vi "read_ini_AdditionalSoftLimits.vi"(8 "error in (no error)":errorcluster caption="错误输入（无错误）", 10 "file ref in":T1, 11 "MotorSystem 输入":refnum<class "MotorSystem.lvclass">) -> (0 "error out":errorcluster caption="错误输出", 2 "file ref out":T1, 3 "MotorSystem 输出":refnum<class "MotorSystem.lvclass">)   [LabVIEW 2016, in "MotionControl.lvlib" / "MotorSystem.lvclass"]
uses:
  <userlib>/MotionControl/MotorSystem/MotorSystem.lvclass
  <vilib>/Utility/config.llb/Config Data RefNum.ctl
  <userlib>/MotionControl/MotorSystem/MotorSystem.lvclass/MotorSystem.ctl
  <vilib>/Utility/config.llb/Read Key (I32).vi
  <vilib>/Utility/config.llb/Read Key (String).vi
  <vilib>/Utility/config.llb/Read Key (Double).vi
  <vilib>/Utility/config.llb/NI_LVConfig.lvlib
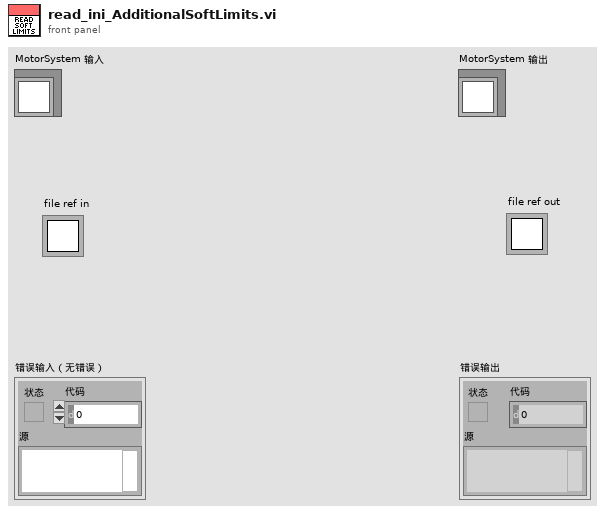
[diagram p1: front panel]
types:
  T1 = typedef "NI_LVConfig.lvlib/Config Data RefNum.ctl" = refnum<k1>
  T2 = cluster{"value":string, cluster{"value":dbl, "value":dbl}}
  T3 = cluster{cluster{"value":string, cluster{"value":dbl, "value":dbl}}[]}
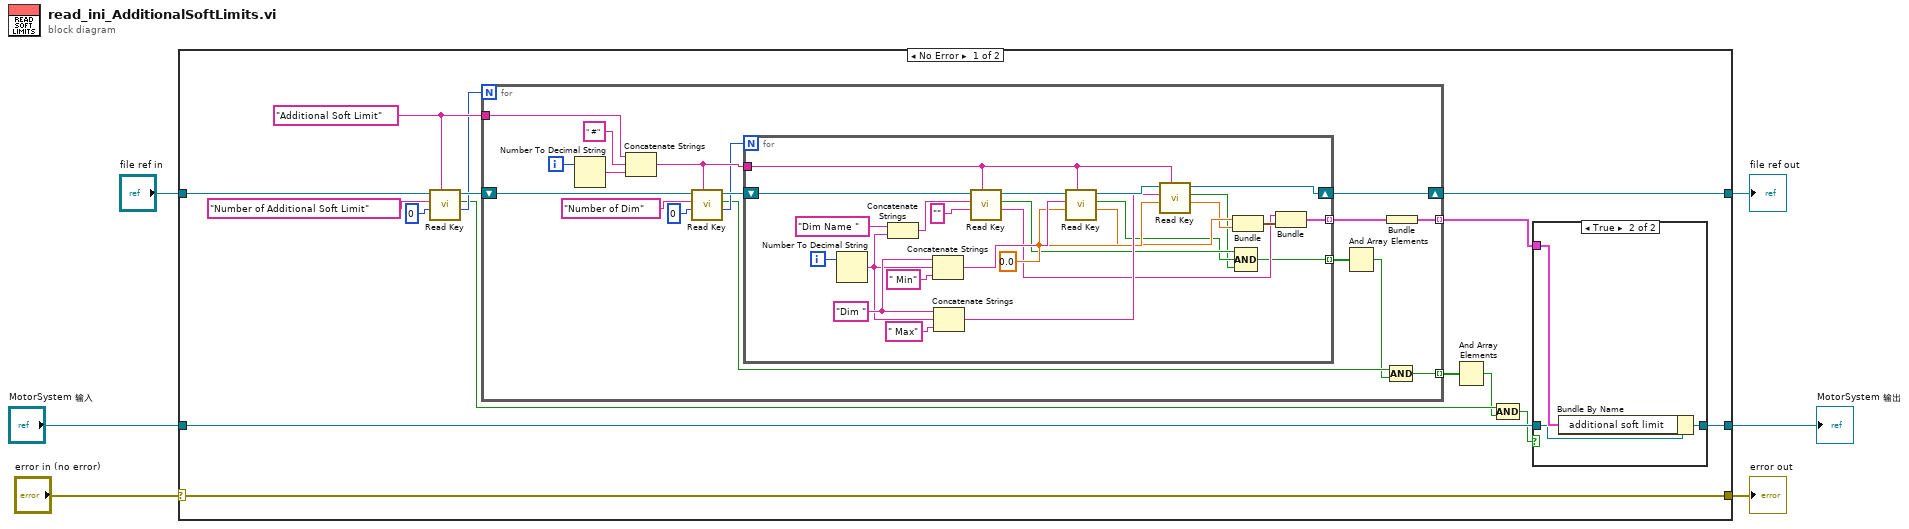
[diagram p0: block diagram]
diagram:
  n1 = case shown="No Error" "error in (no error)" {
    selector: "error in (no error)" -> [w21 w70]
    tunnel: [w21 w70] -> w5
    tunnel: [w11 w69] -> w3
    tunnel: "MotorSystem 输入" -> [w12 w69]
    tunnel: "file ref in" -> [w20 w68]
    tunnel: [w16 w68] -> w1
    frame No Error {
      w18 = "Additional Soft Limit"
      n2 = call-poly <vilib>:"Read Key.vi"("section"=w18, "default value"=0, "key"="Number of Additional Soft Limit", "refnum"=w20) -> ("value"=w14:i32, "found?"=w9:bool, "refnum out"=w17:T1)  [unwired: 4 in, 1 out]
      n3 = for {
        N: w14 -> [_]
        tunnel: w18 -> [w42]
        shift-right: [w34] -> w16
        shift-left: w17 -> [w38]
        tunnel: [w30] -> w13 mode=indexing
        tunnel: [w26] -> w10 mode=indexing
        i -> [w39]
        n4 = Number To Decimal String(number=w39) -> (decimal integer string=w40:string)  [unwired: 1 in]
        n5 = Concatenate Strings(w42, " #", w40) -> (w35:string)
        n6 = call-poly <vilib>:"Read Key.vi"("section"=w35, "default value"=0, "key"="Number of Dim", "refnum"=w38) -> ("value"=w32:i32, "found?"=w28:bool, "refnum out"=w37:T1)  [unwired: 4 in, 1 out]
        n7 = for {
          N: w32 -> [_]
          shift-right: [w54] -> w34
          shift-left: w37 -> [w67]
          tunnel: w35 -> [w55]
          tunnel: [w47] -> w31 mode=indexing
          tunnel: [w43] -> w29 mode=indexing
          i -> [w66]
          w52 = 0.0
          w59 = "Dim "
          n8 = Number To Decimal String(number=w66) -> (decimal integer string=w58:string)  [unwired: 1 in]
          n9 = Concatenate Strings("Dim Name ", w58) -> (w64:string)
          n10 = Concatenate Strings(w59, w58, " Min") -> (w61:string)
          n11 = Concatenate Strings(w59, w58, " Max") -> (w56:string)
          n12 = call-poly <vilib>:"Read Key.vi"("section"=w55, "default value"="", "key"=w64, "refnum"=w67) -> ("value"=w48:string, "found?"=w46:bool, "refnum out"=w63:T1)  [unwired: 4 in, 1 out]
          n13 = call-poly <vilib>:"Read Key.vi"("section"=w55, "default value"=w52, "key"=w61, "refnum"=w63) -> ("value"=w51:dbl, "found?"=w45:bool, "refnum out"=w60:T1)  [unwired: 4 in, 1 out]
          n14 = call-poly <vilib>:"Read Key.vi"("section"=w55, "default value"=w52, "key"=w56, "refnum"=w60) -> ("value"=w50:dbl, "found?"=w44:bool, "refnum out"=w54:T1)  [unwired: 4 in, 1 out]
          n15 = Bundle("value"=w51, "value"=w50) -> (w49:cluster{"value":dbl, "value":dbl})  [unwired: 1 in]
          n16 = Compound Arithmetic op=AND(w46, w45, w44) -> (w43:bool)
          n17 = Bundle("value"=w48, w49) -> (w47:T2)  [unwired: 1 in]
        }
        n18 = And Array Elements(Boolean array=w29) -> (logical AND=w27:bool)
        n19 = Bundle(w31) -> (w30:T3)  [unwired: 1 in]
        n20 = Compound Arithmetic op=AND(w28, w27) -> (w26:bool)
      }
      n21 = And Array Elements(Boolean array=w10) -> (logical AND=w8:bool)
      n22 = Compound Arithmetic op=AND(w9, w8) -> (w7:bool)
      n23 = case shown="True" w7 {
        tunnel: w13 -> [_ w25]
        tunnel: w12 -> [w22 w24]
        tunnel: [w22 w23] -> w11
        frame False {
        }
        frame True {
          n24 = Bundle By Name(cluster=w24, "additional soft limit"=w25) -> (w23:refnum<class "MotorSystem.lvclass">)
        }
      }
    }
    frame Error {
    }
  }
  "error out" <- w5
  "MotorSystem 输出" <- w3
  "file ref out" <- w1
